vi "Mapping Merge Real Positions.vi"(0 "Live Data In":dbl[][](array[numeric]), 5 "X in (1D)":dbl[](array[numeric]), 7 "Y in (1D)":dbl[](array[numeric])) -> (4 "Live Data Out":dbl[][](array[numeric]))   [LabVIEW 2010]
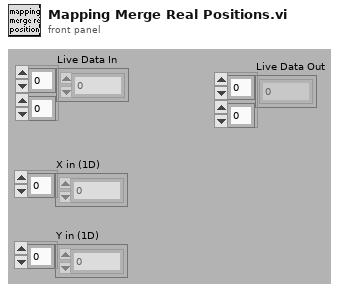
[diagram p1: front panel]
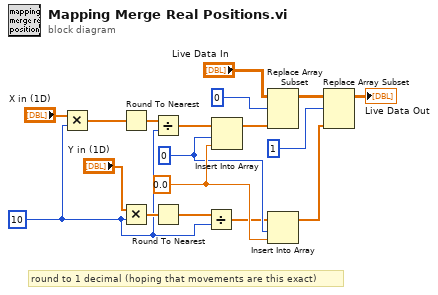
[diagram p0: block diagram]
diagram:
  w3 = i16 10 ("y")
  w17 = 0 ("index")
  w18 = 0.0 ("new element/subarray")
  # "round to 1 decimal (hoping that movements are this exact)"
  n1 = Multiply(x="X in (1D)", y=w3) -> (x*y=w7:dbl[])
  n2 = Round To Nearest(number=w7) -> (nearest integer value=w4:dbl[])
  n3 = Multiply(x="Y in (1D)", y=w3) -> (x*y=w6:dbl[])
  n4 = Divide(x=w4, y=w3) -> (x/y=w2:dbl[])
  n5 = Round To Nearest(number=w6) -> (nearest integer value=w5:dbl[])
  n6 = Divide(x=w5, y=w3) -> (x/y=w1:dbl[])
  n7 = Insert Into Array(array=w2, index=w17, new element=w18) -> (w11:dbl[])
  n8 = Replace Array Subset(array="Live Data In", new element=w11, index (row)=0) -> (w15:dbl[][])  [unwired: 1 in]
  n9 = Insert Into Array(array=w1, index=w17, new element=w18) -> (w10:dbl[])
  n10 = Replace Array Subset(array=w15, new element=w10, index (row)=1) -> (→"Live Data Out":dbl[][])  [unwired: 1 in]
